vi "Parse-attribute.vi"(8 "error in (no error)":errorcluster, 10 "String in":string, 11 "FieldOffset in":refnum<class "FieldOffset.lvclass">) -> (0 "error out":errorcluster, 1 "Valid attribute?":bool, 2 "Remaining string":string, 3 "FieldOffset out":refnum<class "FieldOffset.lvclass">)   [LabVIEW 2013, in "HardwareCharacterization.lvlib" / "FieldOffset.lvclass"]
uses:
  FieldOffset.lvclass
  Attributes.ctl
  Attribute-ID.ctl
  Attribute-XML.lvclass/Attribute-XML.ctl
  ID.lvclass/ID.ctl
  Coordinate/Coordinate.lvclass/Coordinate.ctl
  Write Attribute.vi
  Write ID-attribute.vi
  Coordinate/Write X.vi
  Coordinate/Write Y.vi
  Attribute-XML.lvclass
  ID.lvclass
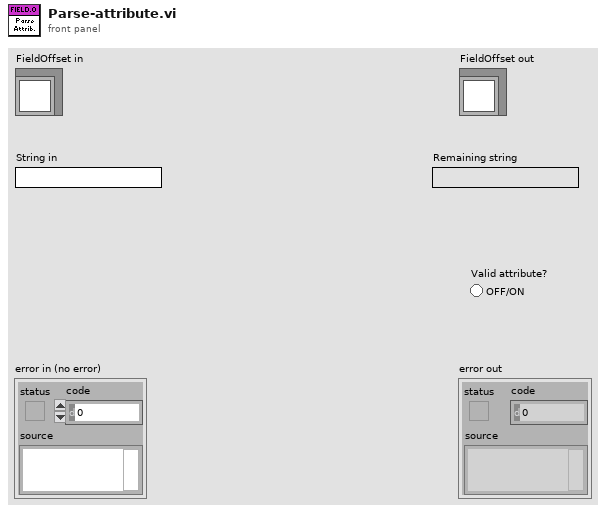
[diagram p1: front panel]
types:
  T1 = typedef "HardwareCharacterization.lvlib/ID.lvclass/Attribute-ID.ctl" = enum16{"FieldOffset", "TransformEnable", "Transform", "Units", "XYCalFactor", "EnableLaser", "JumpDelay", "MarkDelay", "PolyDelay", "LaserOnDelay", "LaserOffDelay", "JumpSpeed", "MarkSpeed", "LaserPowerDelay", "LaserEnableDelay", "LaserPower", "Offset"}
  T2 = typedef "HardwareCharacterization.lvlib/Attribute-XML.lvclass/Attributes.ctl" = enum16{"id"}
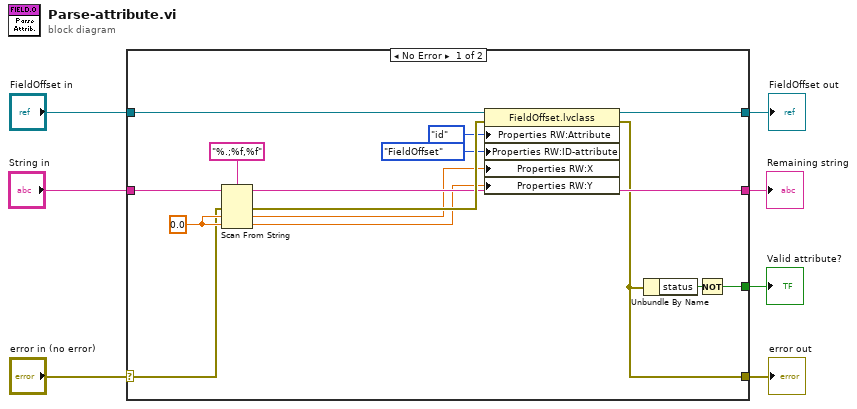
[diagram p0: block diagram]
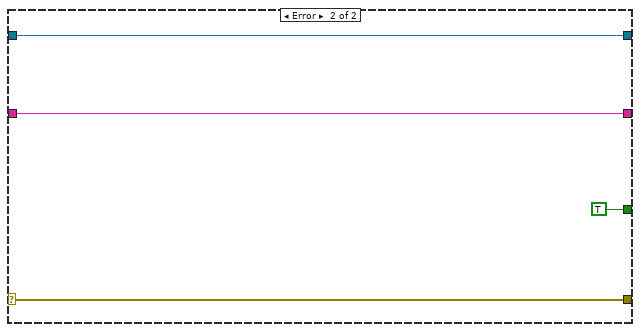
[diagram p2: hidden frame]
diagram:
  n1 = case shown="No Error" "error in (no error)" {
    selector: "error in (no error)" -> [w14 w26]
    tunnel: [w8 w26] -> w6
    tunnel: [w12 w25] -> w4
    tunnel: "FieldOffset in" -> [w17 w25]
    tunnel: "String in" -> [w15 w24]
    tunnel: [w13 w24] -> w2
    tunnel: [w9 TRUE] -> w1
    frame No Error {
      w16 = 0.0 ("default value 2")
      n2 = Scan From String(format string="%.;%f,%f", input string=w15, error in=w14, default 1=w16, default 2=w16) -> (remaining string=w13:string, error out=w20:errorcluster, output 1=w11:dbl, output 2=w10:dbl)  [unwired: 1 in, 1 out]
      n3 = property class="FieldOffset.lvclass"(reference=w17, error in=w20, "Properties RW:Attribute"=Attributes."id" ("Attribute"), "Properties RW:ID-attribute"=Attribute-ID."FieldOffset" ("ID-attribute"), "Properties RW:X"=w11, "Properties RW:Y"=w10) -> (reference out=w12:refnum<class "FieldOffset.lvclass">, error out=w8:errorcluster)
      n4 = Unbundle By Name(w8) -> ("status"=w21:bool)
      n5 = Not(x=w21) -> (.not. x?=w9:bool)
    }
    frame Error {
    }
  }
  "error out" <- w6
  "FieldOffset out" <- w4
  "Remaining string" <- w2
  "Valid attribute?" <- w1
